vi "HK Channel Get Formatted Value Table.vi"(8 "error in (no error)":errorcluster, 11 "HK Table in":refnum<class "HK Table.lvclass">) -> (0 "error out":errorcluster, 1 "Hdr":string[](array[string]), 2 "Table":string[][](array[string]), 3 "HK Table out":refnum<class "HK Table.lvclass">, 5 "Values":dbl[](array[numeric]))   [LabVIEW 2024, in "HK Table.lvclass"]
uses:
  HK Table.lvclass
  HK Table.lvclass/HK Table.ctl
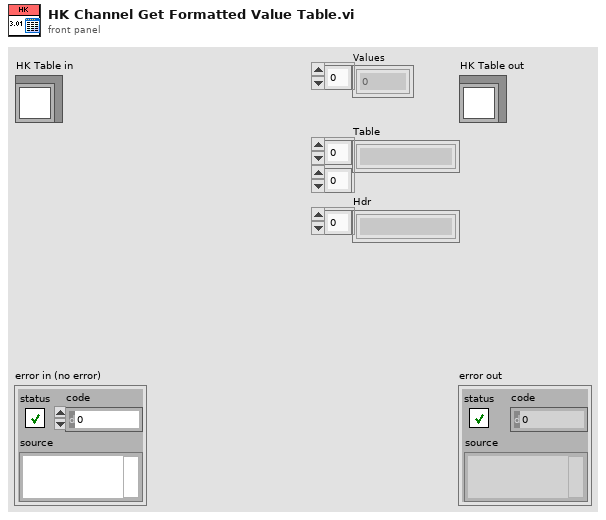
[diagram p1: front panel]
types:
  T1 = typedef "HK Table.lvclass/HK Current Value Table Element.ctl" = cluster{"Value":dbl, "Time Stamp":timestamp, "Running Avg.":dbl, "Std. Dev.":dbl, "Recent Values":dbl[], "Timestamps":timestamp[], "Alarm Status":T2}
  T2 = typedef "HK Item.lvclass/HK Alarm enum Status.ctl" = enum16{"No Alarm", "Red Low", "Red High", "Yellow Low", "Yellow High"}
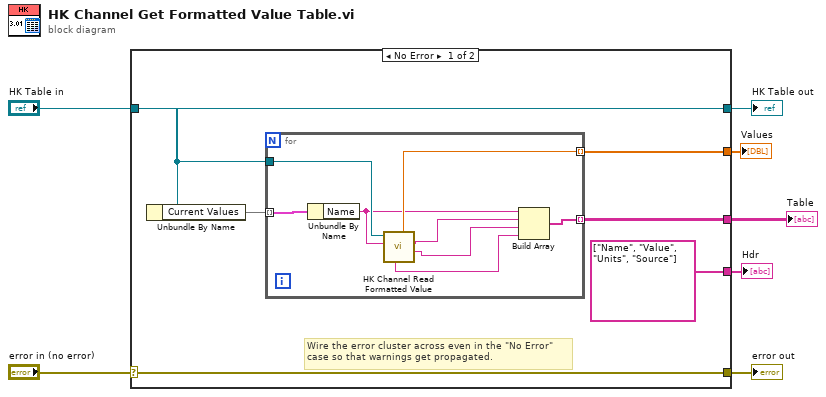
[diagram p0: block diagram]
diagram:
  n1 = case shown="No Error" "error in (no error)" {
    selector: "error in (no error)" -> [w13 w23]
    tunnel: [w13 w23] -> w6
    tunnel: [w11 w22] -> w4
    tunnel: "HK Table in" -> [w11 w22]
    tunnel: [w10 _] -> w3
    tunnel: [string[] ["Name", "Value", "Units", "Source"] _] -> w2
    tunnel: [w8 _] -> w1
    frame No Error {
      # "Wire the error cluster across even in the \"No Error\"\ncase so that warnings get propagated."
      n2 = Unbundle By Name(w11) -> ("Current Values"=w12:map{string, T1})
      n3 = for {
        tunnel: w12 -> [w21] mode=indexing
        tunnel: w11 -> [w19]
        tunnel: [w20] -> w10 mode=indexing
        tunnel: [w18] -> w8 mode=indexing
        n4 = Unbundle By Name(w21) -> ("Name"=w17:string)
        n5 = call-dynamic "HK Channel Read Formatted Value.vi"("Name"=w17, "HK Table.lvclass"=w19) -> ("Units"=w15:string, "Value Formatted"=w14:string, "Value"=w18:dbl, "Source"=w16:string)  [unwired: 2 in, 4 out]
        n6 = Build Array(w17, w14, w15, w16) -> (w20:string[])
      }
    }
    frame Error {
    }
  }
  "error out" <- w6
  "HK Table out" <- w4
  "Table" <- w3
  "Hdr" <- w2
  "Values" <- w1
